vi "Main.vi"() -> ()   [LabVIEW 2025]
doc: "Use this template to build a simple state machine design pattern. Each state executes code and determines which state to transition to."
uses:
  controls/State.ctl
  controls/Data.ctl
panel:
  in  "Period":dbl=100.0
  in  "Amplitude":dbl=1.0
  out "Waveform Chart":dbl(graph)
  in  "Waveform Type":i32(knob) min=0 max=2 step=1 scale=0.0..2.0
  in  "Start/Stop":bool
  in  "Exit":bool
  # "Signal Generator"
  # "Wave Setup"
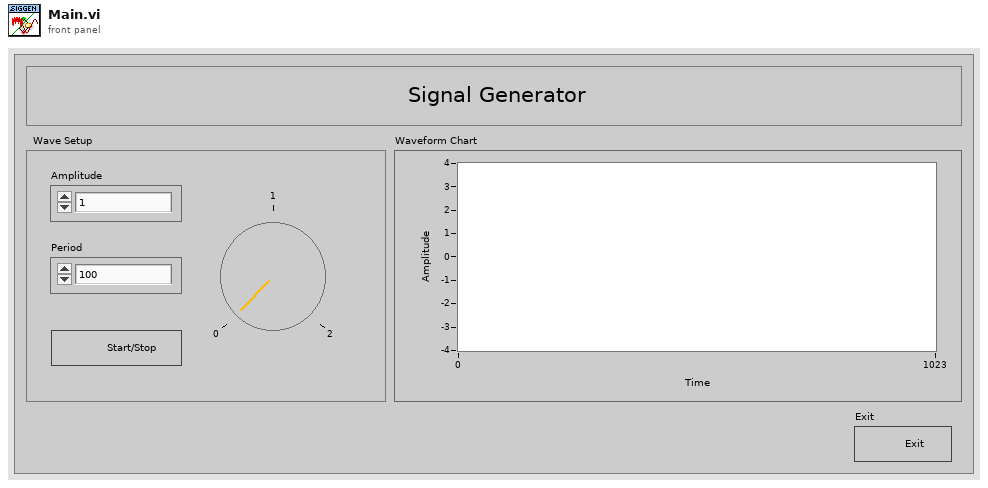
[diagram p1: front panel]
types:
  T1 = typedef "Data.ctl" = cluster{"Amplitude":dbl, "Current Data":dbl, "Period":dbl, "Index":i32}
  T2 = typedef "State.ctl" = enum16{"Initialize", "Wait for Event", "Sine", "Square", "Triangular", "Graph", "Exit"}
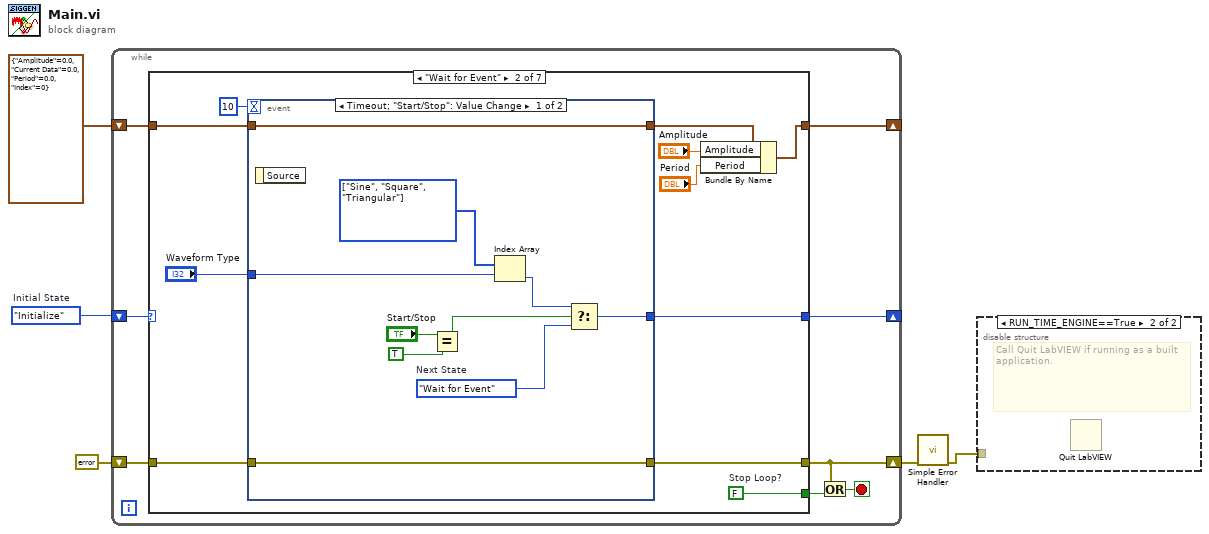
[diagram p0: block diagram]
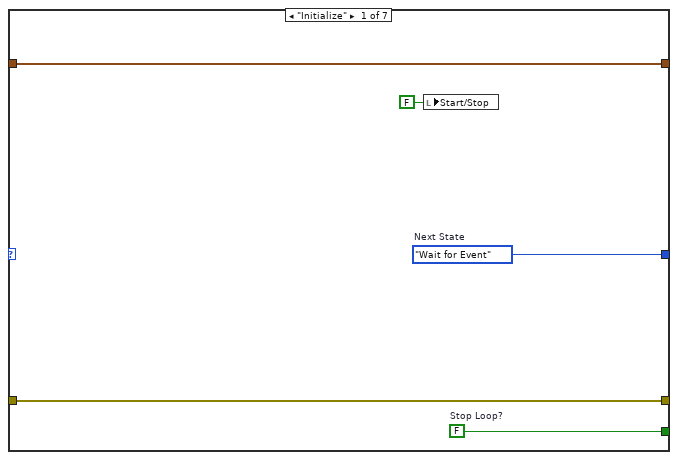
[diagram p3: hidden frame]
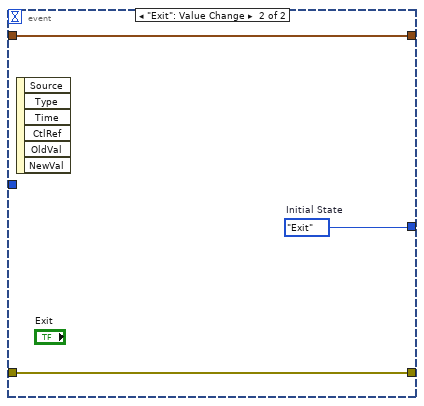
[diagram p4: hidden frame]
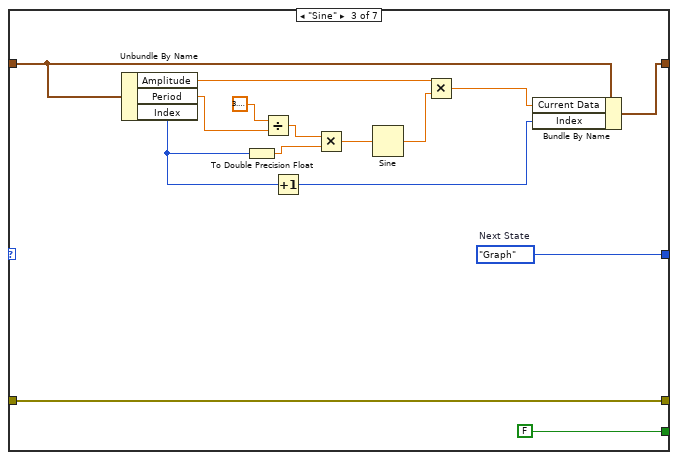
[diagram p5: hidden frame]
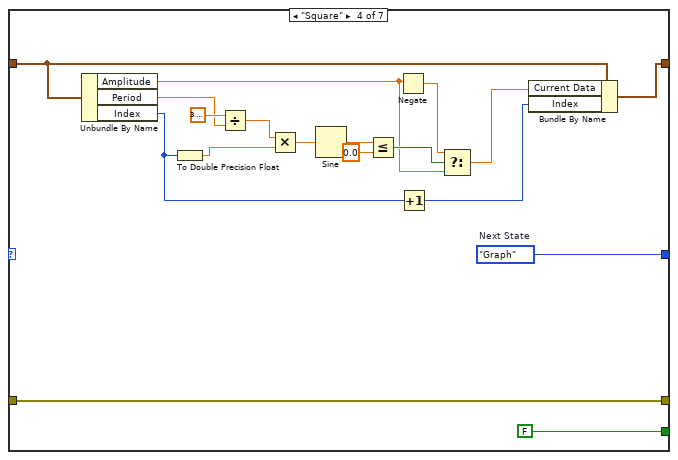
[diagram p6: hidden frame]
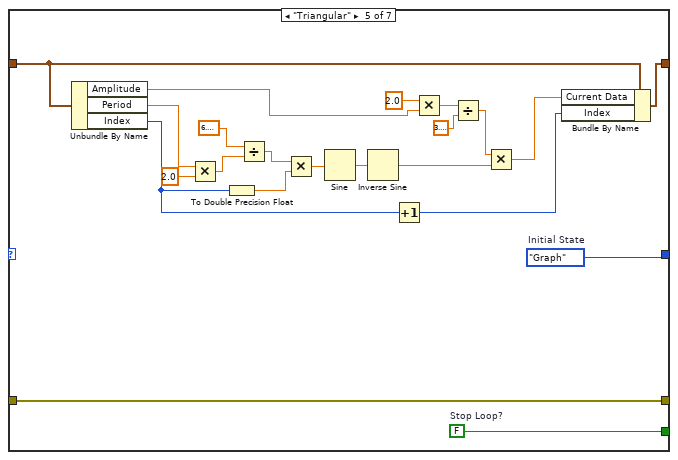
[diagram p7: hidden frame]
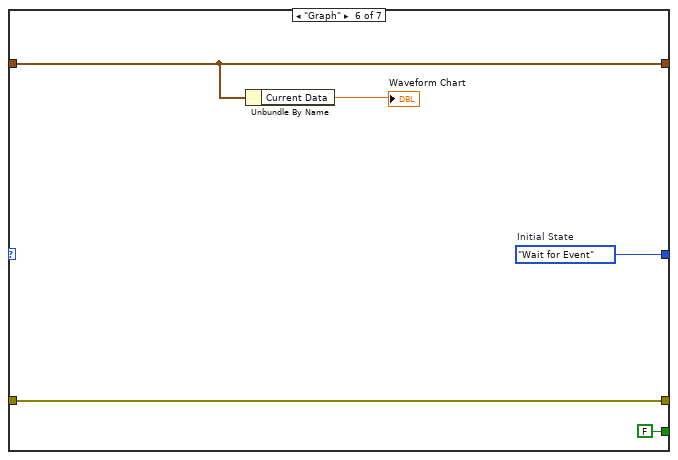
[diagram p8: hidden frame]
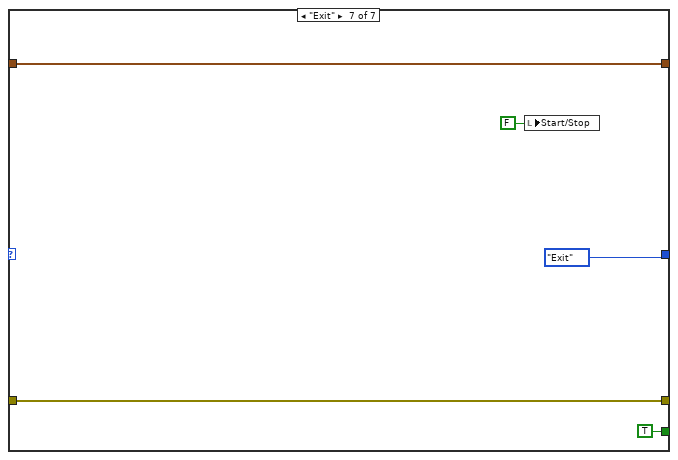
[diagram p9: hidden frame]
diagram:
  w1 = State."Initialize"  # Initial State
  n1 = while {
    shift-right: [w12] -> _
    shift-left: T1 {"Amplitude"=0.0, "Current Data"=0.0, "Period"=0.0, "Index"=0} ("Data") -> [w13]
    shift-right: [w8] -> w3
    shift-left: errorcluster {"status"=FALSE, "code"=0, "source"=""} ("error constant") -> [w11]
    shift-right: [w7] -> _
    shift-left: w1 -> [w6]
    stop <- w9 stop-if-true
    # "Main VI State Machine"
    n2 = case shown="\"Wait for Event\"" w6 {
      tunnel: [w14 w23 w57 w75 w95 w98 State."Exit" ("Initial State")] -> w7
      tunnel: [w18 w29 FALSE ("Stop Loop?") FALSE ("Stop Loop?") w97 FALSE ("Stop Loop?") TRUE ("Stop Loop?")] -> w10
      tunnel: w13 -> [w16 w28 w46 w62 w80 w101 w107]
      tunnel: [w16 w21 w45 w61 w79 w101 w107] -> w12
      tunnel: w11 -> [w17 w27 w55 w73 w96 w102 w106]
      tunnel: [w17 w26 w55 w73 w96 w102 w106] -> w8
      frame "Initialize" {
        w18 = FALSE  # Stop Loop?
        w14 = State."Wait for Event"  # Next State
        # "Initialize - Initialize the application."
        n3 = local write "Start/Stop"(FALSE ("Start/Stop")) -> ()
      }
      frame "Wait for Event" {
        w29 = FALSE  # Stop Loop?
        # "Wait for Event - Use an Event Structure to monitor the user interface for events that run different states of the state machine."
        n4 = event shown="[0] Timeout;  \"Start/Stop\": Value Change" {
          selector: _ -> [_ _]
          dyn-events: _ -> [_ _]
          timeout: 10 -> [_ _]
          tunnel: [w30 w40] -> w23
          tunnel: w28 -> [w39 w42]
          tunnel: [w39 w42] -> w22
          tunnel: w27 -> [w38 w41]
          tunnel: [w38 w41] -> w26
          tunnel: "Waveform Type" -> [w33 _]
          event Timeout; "Start/Stop": Value Change {
            w31 = T2[] [enum."Sine", enum."Square", enum."Triangular"] items=["Initialize", "Wait for Event", "Sine", "Square", "Triangular", "Graph", "Exit"]
            w37 = State."Wait for Event"  # Next State
            n5 = event-data() -> ()  [unwired: 1 in, 1 out]
            n6 = Equal?(x="Start/Stop", y=TRUE) -> (x = y?=w34:bool)
            n7 = Index Array(array=w31, index=w33) -> (element=w32:T2)
            n8 = Select(t=w32, s=w34, f=w37) -> (s? t:f=w30:T2)
          }
          event "Exit": Value Change {
            w40 = State."Exit"  # Initial State
            n9 = event-data() -> ()  [unwired: 1 in, 6 out]
          }
        }
        n10 = Bundle By Name(cluster=w22, "Amplitude"="Amplitude", "Period"="Period") -> (w21:T1)
      }
      frame "Sine" {
        w57 = State."Graph"  # Next State
        # "User State 1 - Replace this state with functionality for your own application."
        n11 = Unbundle By Name(w46) -> ("Amplitude"=w54:dbl, "Period"=w51:dbl, "Index"=w47:i32)
        n12 = To Double Precision Float(number=w47) -> (double precision float=w48:dbl)
        n13 = Divide(x=3.141592653589793, y=w51) -> (x/y=w49:dbl)
        n14 = Increment(x=w47) -> (x+1=w43:i32)
        n15 = Multiply(x=w49, y=w48) -> (x*y=w50:dbl)
        n16 = Sine(x=w50) -> (sin(x)=w53:dbl)
        n17 = Multiply(x=w54, y=w53) -> (x*y=w44:dbl)
        n18 = Bundle By Name(cluster=w46, "Current Data"=w44, "Index"=w43) -> (w45:T1)
      }
      frame "Square" {
        w75 = State."Graph"  # Next State
        # "User State 2 - Replace this state with functionality for your own application."
        n19 = Unbundle By Name(w62) -> ("Amplitude"=w63:dbl, "Period"=w71:dbl, "Index"=w59:i32)
        n20 = To Double Precision Float(number=w59) -> (double precision float=w69:dbl)
        n21 = Divide(x=3.141592653589793, y=w71) -> (x/y=w70:dbl)
        n22 = Multiply(x=w70, y=w69) -> (x*y=w68:dbl)
        n23 = Sine(x=w68) -> (sin(x)=w67:dbl)
        n24 = Less Or Equal?(x=w67, y=0.0) -> (x <= y?=w65:bool)
        n25 = Negate(x=w63) -> (-x=w64:dbl)
        n26 = Increment(x=w59) -> (x+1=w58:i32)
        n27 = Select(t=w64, s=w65, f=w63) -> (s? t:f=w60:dbl)
        n28 = Bundle By Name(cluster=w62, "Current Data"=w60, "Index"=w58) -> (w61:T1)
      }
      frame "Triangular" {
        w95 = State."Graph"  # Initial State
        w97 = FALSE  # Stop Loop?
        # "Exit - Exit the application."
        n29 = Unbundle By Name(w80) -> ("Amplitude"=w81:dbl, "Period"=w94:dbl, "Index"=w76:i32)
        n30 = Multiply(x=w94, y=2.0) -> (x*y=w93:dbl)
        n31 = To Double Precision Float(number=w76) -> (double precision float=w89:dbl)
        n32 = Divide(x=6.283185307179586, y=w93) -> (x/y=w91:dbl)
        n33 = Multiply(x=w91, y=w89) -> (x*y=w88:dbl)
        n34 = Sine(x=w88) -> (sin(x)=w87:dbl)
        n35 = Inverse Sine(1:w87) -> (0:w86:dbl)
        n36 = Increment(x=w76) -> (x+1=w77:i32)
        n37 = Multiply(x=2.0, y=w81) -> (x*y=w85:dbl)
        n38 = Divide(x=w85, y=3.141592653589793) -> (x/y=w83:dbl)
        n39 = Multiply(x=w83, y=w86) -> (x*y=w78:dbl)
        n40 = Bundle By Name(cluster=w80, "Current Data"=w78, "Index"=w77) -> (w79:T1)
      }
      frame "Graph" {
        w98 = State."Wait for Event"  # Initial State
        n41 = Unbundle By Name(w101) -> ("Current Data"=→"Waveform Chart":dbl)
      }
      frame "Exit" {
        n42 = local write "Start/Stop"(FALSE ("Start/Stop")) -> ()
      }
    }
    n43 = Or(x=w8, y=w10) -> (x .or. y?=w9:bool)
  }
  n44 = call <vilib>:"Simple Error Handler.vi"("error in (no error)"=w3) -> ("error out"=w2:errorcluster)  [unwired: 4 in, 4 out]
  n45 = disable-structure shown="RUN_TIME_ENGINE==True" {
    disable-tunnel: w2 -> [_ _]
    frame condition #0 (active) {
    }
    frame condition #1 {
      # "Call Quit LabVIEW if running as a built application."
      n46 = Quit LabVIEW() -> ()  [unwired: 1 in]
    }
  }
